vi "Demonstration of k-means assumptions.vi"() -> ()   [LabVIEW 2020]
doc: "This example is meant to illustrate situations where k-means will produce unintuitive and possibly unexpected clusters. In the first three plots, the input data does not conform to some implicit assumption that k-means makes and undesirable clusters are produced as a result. In the last plot, k-means returns intuitive clusters despite unevenly sized blobs."
uses:
  Model/Unsupervised/Cluster/KMeans/KMeans.lvclass
  C:/Users/cipop/TDF Dropbox/2_Technologies de France/1 - Services et Etudes/PLAIY/2 - DEV/PLAIYLAB/code/Model/Model.lvclass
  Model/Unsupervised/Cluster/KMeans/Controls/kmeans_params.ctl
  Display/Classification/2D/Predicted/Controls/PredictedParameter.ctl
  Display/_Controls/Style.ctl
  <vilib>/Analysis/baseanly.llb/Real A x B.vi
  Model/Unsupervised/Cluster/KMeans/KMeans.vi
  <vilib>/Analysis/Matrix/Numeric/Conversions/Array To Matrix - RA2.vi
  <vilib>/Analysis/Matrix/Numeric/Conversions/Matrix To Array - RM.vi
  <vilib>/Analysis/Matrix/NI_Matrix.lvlib
  <vilib>/Analysis/NI_AALBase.lvlib
panel:
  in  "Local":T1
  in  "error in (no error)":errorcluster caption="entrée d'erreur (pas d'erreur)"
  out "error out":errorcluster
  out "Plot 4":cluster{"X":dbl[], "Y":dbl[]}[](graph) caption="Unevenly Sized Blobs"
  out "Plot 3":cluster{"X":dbl[], "Y":dbl[]}[](graph) caption="Unequal Variance"
  out "Plot 2":cluster{"X":dbl[], "Y":dbl[]}[](graph) caption="Anisotropicly Distributed Blobs"
  out "Plot":cluster{"X":dbl[], "Y":dbl[]}[](graph) caption="Incorrect Number of Blobs"
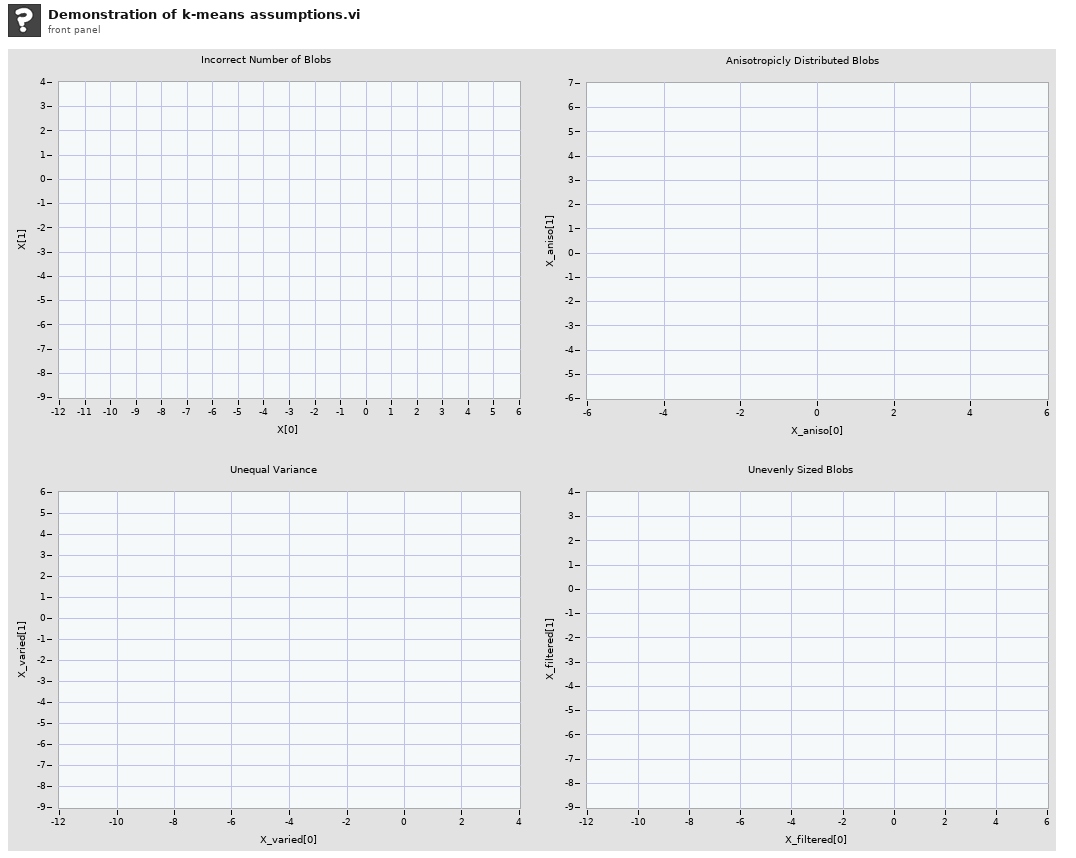
[diagram p1: front panel]
types:
  T1 = cluster{"X":dbl[][], "y":dbl[], "varied":dbl[][], "KMeans":refnum<class "KMeans.lvclass">}
  T2 = cluster{"n_samples":i32[], "n_features":u32, "centers":i32[][], "cluster_std":dbl[], "centermin":dbl, "centermax":dbl, "shuffle":bool, "random_state":i32, "Returns":string}
  T3 = typedef "Style.ctl" = enum16{"Empty circle", "Full circle", "Empty square", "Full square", "Cross"}
  T4 = typedef "PredictedParameter.ctl" = cluster{"Plot":refnum<vi>, "Data":cluster{"X":dbl[][], "Predict":dbl[][]}, "Indexe":cluster{"X":i32, "Y":i32}, "Point Property":cluster{"Style":T3, "Label Color":u32[]}}
  T5 = typedef "kmeans_params.ctl" = cluster{"n_clusters":dbl, "init":cluster{"init_type":string, "init_list":dbl[][]}, "n_init":dbl, "max_iter":dbl, "tol":dbl, "verbose":dbl, "random_state":dbl, "copy_x":bool, "algorithm":string}
  T6 = cluster{" 4DArray":cluster{"1":string[][], "2":string[][]}[], " 3DArray":cluster{"Tableau":string[][]}[], "Sparse Matrix 2DArray":string[][], " 2DArray":string[][], " 1DArray":string[]}
  T7 = typedef "NI_Matrix.lvlib/RealMatrix.ctl" = dbl[][]
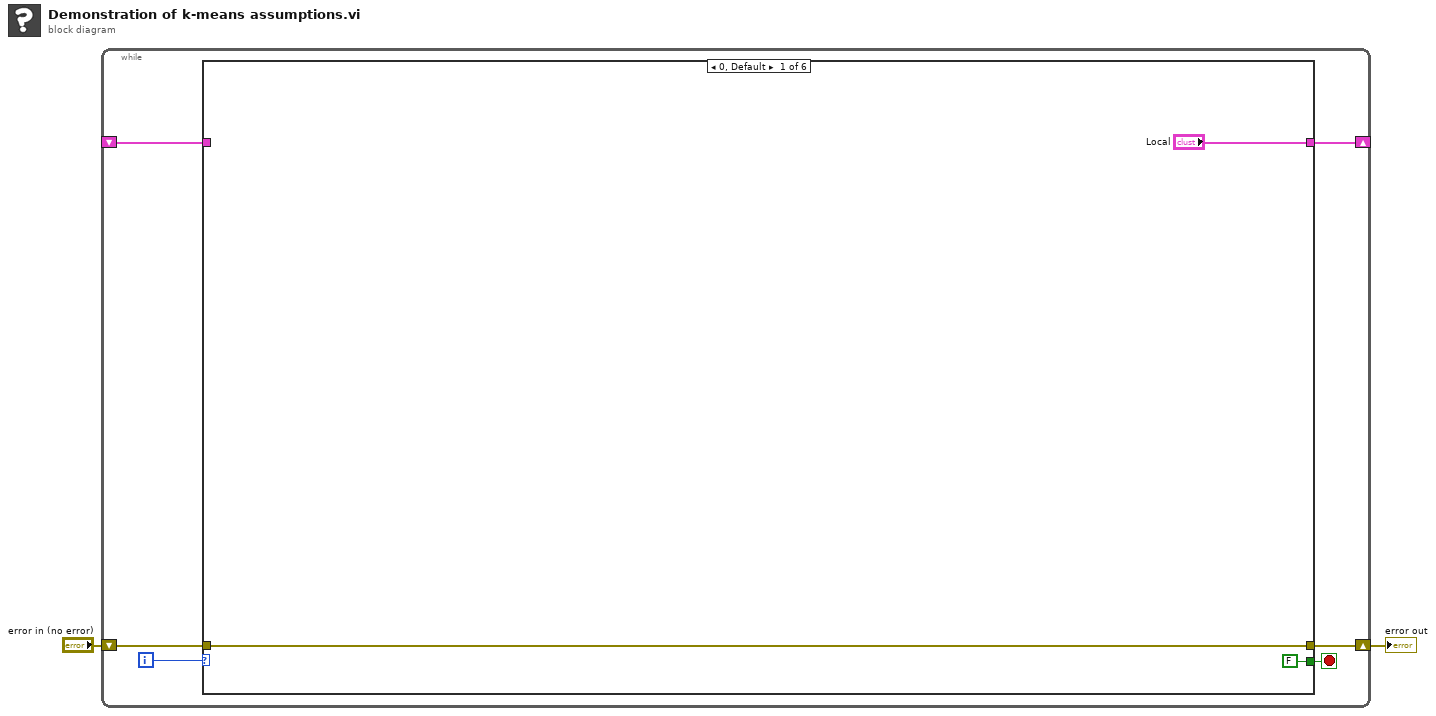
[diagram p0: block diagram]
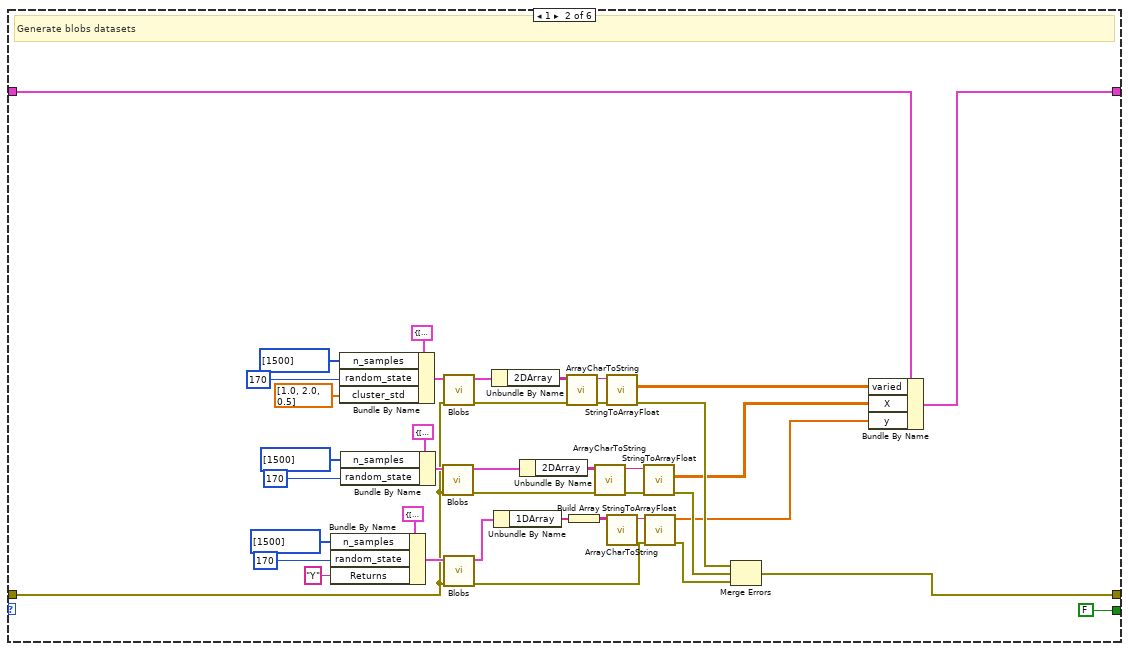
[diagram p2: hidden frame]
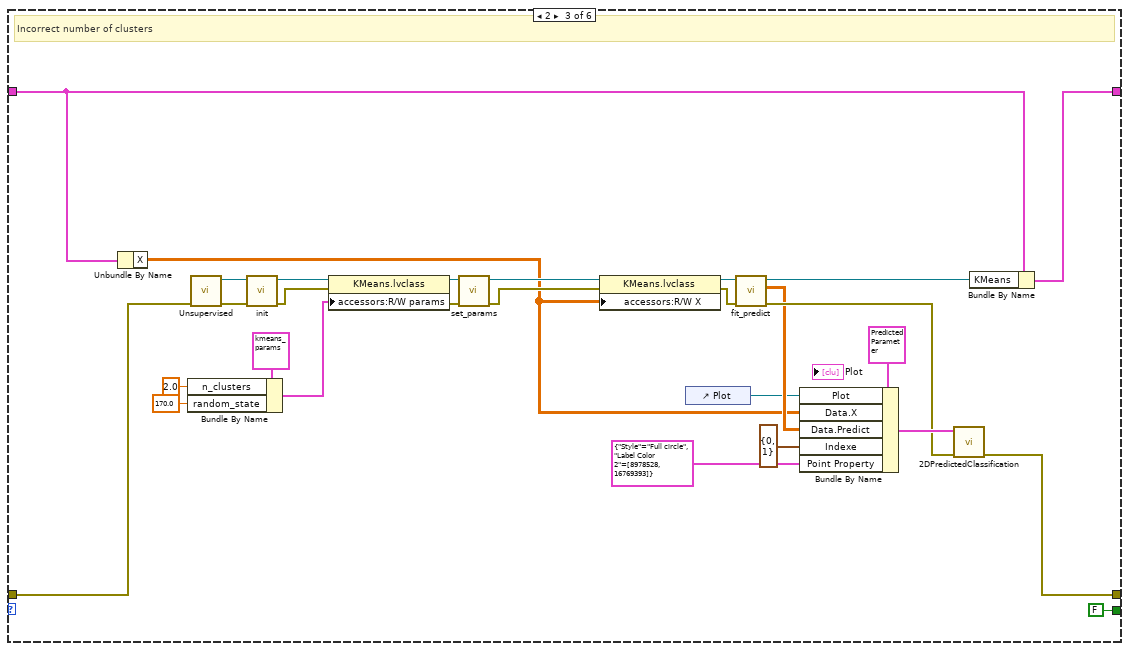
[diagram p3: hidden frame]
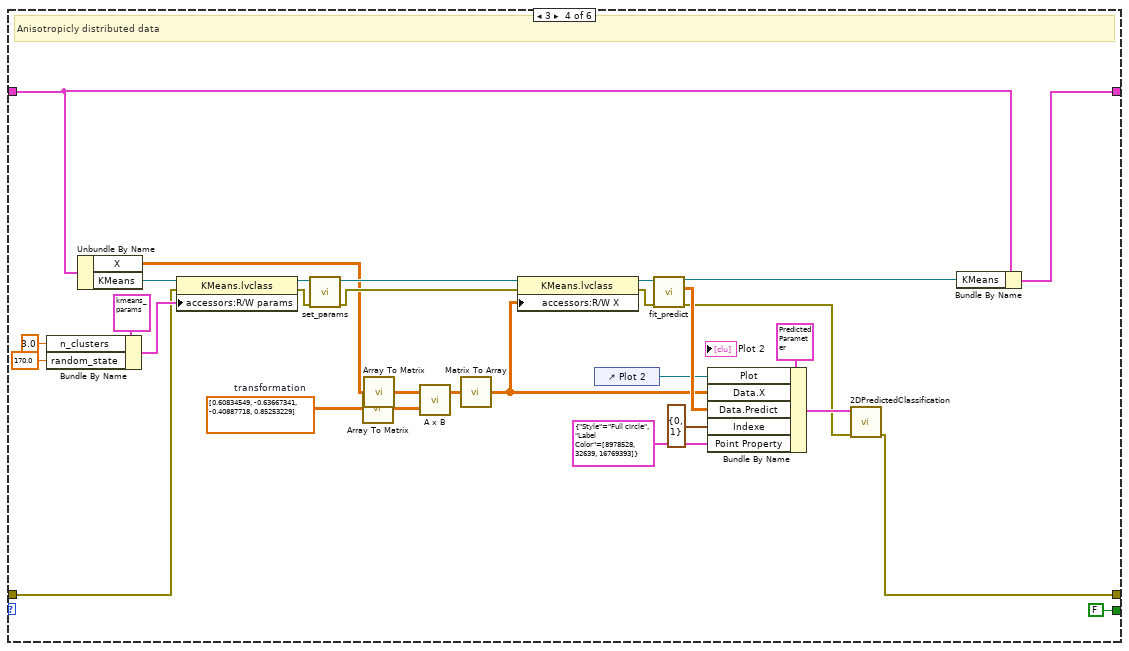
[diagram p4: hidden frame]
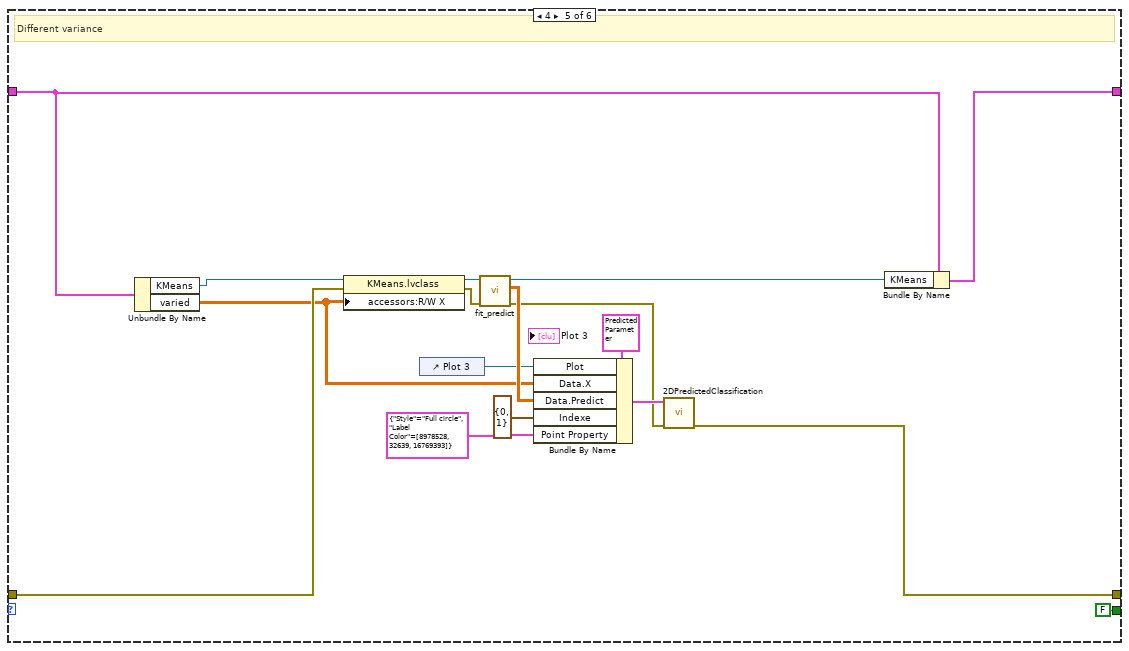
[diagram p5: hidden frame]
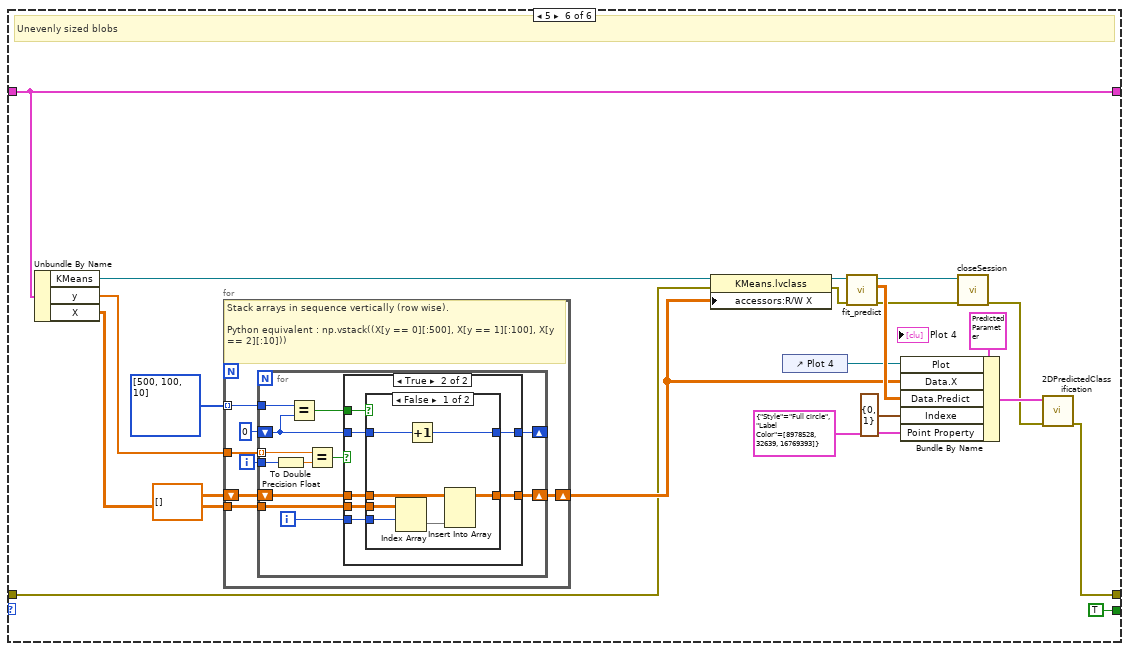
[diagram p6: hidden frame]
diagram:
  n1 = while {
    shift-right: [w6] -> w1
    shift-left: "error in (no error)" -> [w7]
    shift-right: [w4] -> _
    shift-left: _ -> [w3]
    i -> [w8]
    stop <- w5 stop-if-true
    n2 = case shown="0, Default" w8 {
      tunnel: w7 -> [w10 w19 w56 w86 w116 w132]
      tunnel: [w10 w29 w57 w90 w115 w131] -> w6
      tunnel: [FALSE FALSE FALSE FALSE FALSE TRUE] -> w5
      tunnel: ["Local" w15 w51 w79 w110 w125] -> w4
      tunnel: w3 -> [_ w16 w52 w81 w111 w125]
      frame 0, Default {
      }
      frame 1 {
        # "Generate blobs datasets"
        n3 = Bundle By Name(cluster=T2 {"n_samples"=[100], "n_features"=2, "centers"=[], "cluster_std"=[1.0], "centermin"=-10.0, "centermax"=10.0, "shuffle"=TRUE, "random_state"=-1, "Returns"="X"} ("make_blobs"), "n_samples"=i32[] [1500], "random_state"=170, "Returns"="Y") -> (w38:T2)
        n4 = Bundle By Name(cluster=T2 {"n_samples"=[100], "n_features"=2, "centers"=[], "cluster_std"=[1.0], "centermin"=-10.0, "centermax"=10.0, "shuffle"=TRUE, "random_state"=-1, "Returns"="X"} ("make_blobs"), "n_samples"=i32[] [1500], "random_state"=170, "cluster_std"=dbl[] [1.0, 2.0, 0.5]) -> (w21:T2)
        n5 = Bundle By Name(cluster=T2 {"n_samples"=[100], "n_features"=2, "centers"=[], "cluster_std"=[1.0], "centermin"=-10.0, "centermax"=10.0, "shuffle"=TRUE, "random_state"=-1, "Returns"="X"} ("make_blobs"), "n_samples"=i32[] [1500], "random_state"=170) -> (w49:T2)
        n6 = call "Blobs.vi"("error in (no error)"=w19, "make_blobs"=w49) -> ("error out"=w42:errorcluster, "Data"=w45:T6)  [unwired: 8 in]
        n7 = call "Blobs.vi"("error in (no error)"=w19, "make_blobs"=w21) -> ("error out"=w28:errorcluster, "Data"=w25:T6)  [unwired: 8 in]
        n8 = call "Blobs.vi"("error in (no error)"=w19, "make_blobs"=w38) -> ("error out"=w33:errorcluster, "Data"=w34:T6)  [unwired: 8 in]
        n9 = Unbundle By Name(w25) -> ("2DArray"=w27:string[][])
        n10 = Unbundle By Name(w34) -> ("1DArray"=w36:string[])
        n11 = Unbundle By Name(w45) -> ("2DArray"=w43:string[][])
        n12 = call "ArrayCharToString.vi"("TAB"=w27) -> ("Instruction"=w26:string)  [unwired: 10 in]
        n13 = Build Array(w36) -> (w32:string[][])
        n14 = call "ArrayCharToString.vi"("TAB"=w43) -> ("Instruction"=w44:string)  [unwired: 10 in]
        n15 = call "StringToArrayFloat.vi"("entrée d'erreur (pas d'erreur)"=w28, "Return value"=w26) -> ("error IO"=w18:errorcluster, "2DArray"=w14:dbl[][])  [unwired: 7 in, 1 out]
        n16 = call "ArrayCharToString.vi"("TAB"=w32) -> ("Instruction"=w35:string)  [unwired: 10 in]
        n17 = call "StringToArrayFloat.vi"("entrée d'erreur (pas d'erreur)"=w42, "Return value"=w44) -> ("error IO"=w30:errorcluster, "2DArray"=w13:dbl[][])  [unwired: 7 in, 1 out]
        n18 = call "StringToArrayFloat.vi"("entrée d'erreur (pas d'erreur)"=w33, "Return value"=w35) -> ("error IO"=w31:errorcluster, "1DArray"=w12:dbl[])  [unwired: 7 in, 1 out]
        n19 = Merge Errors(w18, w30, w31) -> (w29:errorcluster)
        n20 = Bundle By Name(cluster=w16, "varied"=w14, "X"=w13, "y"=w12) -> (w15:T1)
      }
      frame 2 {
        # "Incorrect number of clusters"
        n21 = Unbundle By Name(w52) -> ("X"=w53:dbl[][])
        n22 = Bundle By Name(cluster=T5 {"n_clusters"=8.0, "init"={"init_type"="k-means++", "init_list"=[]}, "n_init"=10.0, "max_iter"=300.0, "tol"=0.0001, "verbose"=0.0, "random_state"=0.0, "copy_x"=TRUE, "algorithm"="auto"} ("R/W params"), "n_clusters"=2.0, "random_state"=170.0) -> (w65:T5)
        n23 = call-poly "Unsupervised.vi"("error in"=w56) -> ("error out"=w70:errorcluster, "out"=w71:refnum<class "KMeans.lvclass">)  [unwired: 9 in]
        n24 = call-dynamic "init.vi"("error in (no error)"=w70, "Model en entrée"=w71) -> ("error out"=w72:errorcluster, "Model en sortie"=w76:refnum<class "KMeans.lvclass">)  [unwired: 8 in]
        n25 = property class="KMeans.lvclass"(reference=w76, error in=w72, "accessors:R/W params"=w65) -> (reference out=w75:refnum<class "KMeans.lvclass">, error out=w77:errorcluster)
        n26 = call-dynamic "set_params.vi"("error in (no error)"=w77, "KMeans.lvclass 2"=w75) -> ("error out"=w73:errorcluster, "KMeans.lvclass"=w74:refnum<class "KMeans.lvclass">)  [unwired: 8 in]
        n27 = property class="KMeans.lvclass"(reference=w74, error in=w73, "accessors:R/W X"=w53) -> (reference out=w67:refnum<class "KMeans.lvclass">, error out=w66:errorcluster)
        n28 = control-ref of="Plot"() -> (w55:refnum<vi>)
        n29 = call-dynamic "fit_predict.vi"("error in (no error)"=w66, "KMeans.lvclass 2"=w67) -> ("error out"=w61:errorcluster, "C"=w60:dbl[][], "KMeans.lvclass"=w50:refnum<class "KMeans.lvclass">)  [unwired: 7 in]
        n30 = Bundle By Name(cluster=T4 {"Plot"=refnum, "Data"={"X"=[], "Predict"=[]}, "Indexe"={"X"=0, "Y"=1}, "Point Property"={"Style"=enum."Full circle", "Label Color"=[8978528, 4367871, 1985280]}} ("Parameters"), "Plot"=w55, "Data.X"=w53, "Data.Predict"=w60, "Indexe"=cluster{"X":i32, "Y":i32} {"X"=0, "Y"=1}, "Point Property"=cluster{"Style":T3, "Label Color 2":u32[]} {"Style"=enum."Full circle", "Label Color 2"=[8978528, 16769393]}) -> (w63:T4)
        n31 = call "2DPredictedClassification.vi"("error in"=w61, "Parameters"=w63) -> ("error out"=w57:errorcluster)  [unwired: 9 in]
        n32 = Bundle By Name(cluster=w52, "KMeans"=w50) -> (w51:T1)
      }
      frame 3 {
        w106 = dbl[][] [[0.60834549, -0.63667341], [-0.40887718, 0.85253229]]  # transformation
        # "Anisotropicly distributed data"
        n33 = Bundle By Name(cluster=T5 {"n_clusters"=8.0, "init"={"init_type"="k-means++", "init_list"=[]}, "n_init"=10.0, "max_iter"=300.0, "tol"=0.0001, "verbose"=0.0, "random_state"=0.0, "copy_x"=TRUE, "algorithm"="auto"} ("R/W params"), "n_clusters"=3.0, "random_state"=170.0) -> (w89:T5)
        n34 = Unbundle By Name(w81) -> ("X"=w82:dbl[][], "KMeans"=w78:refnum<class "KMeans.lvclass">)
        n35 = property class="KMeans.lvclass"(reference=w78, error in=w86, "accessors:R/W params"=w89) -> (reference out=w99:refnum<class "KMeans.lvclass">, error out=w85:errorcluster)
        n36 = call-dynamic "set_params.vi"("error in (no error)"=w85, "KMeans.lvclass 2"=w99) -> ("error out"=w101:errorcluster, "KMeans.lvclass"=w100:refnum<class "KMeans.lvclass">)  [unwired: 8 in]
        n37 = call-poly <vilib>:"Array To Matrix.vi"("Real 2D Array"=w106) -> ("Real Matrix"=w105:T7)
        n38 = call-poly <vilib>:"Array To Matrix.vi"("Real 2D Array"=w82) -> ("Real Matrix"=w107:T7)
        n39 = call-poly <vilib>:"A x B.vi"("B"=w105, "A"=w107) -> ("A x B"=w104:T7)  [unwired: 1 out]
        n40 = call-poly <vilib>:"Matrix To Array.vi"("Real Matrix"=w104) -> ("Real 2D Array"=w83:dbl[][])
        n41 = property class="KMeans.lvclass"(reference=w100, error in=w101, "accessors:R/W X"=w83) -> (reference out=w102:refnum<class "KMeans.lvclass">, error out=w103:errorcluster)
        n42 = control-ref of="Plot 2"() -> (w87:refnum<vi>)
        n43 = call-dynamic "fit_predict.vi"("error in (no error)"=w103, "KMeans.lvclass 2"=w102) -> ("error out"=w91:errorcluster, "C"=w92:dbl[][], "KMeans.lvclass"=w80:refnum<class "KMeans.lvclass">)  [unwired: 7 in]
        n44 = Bundle By Name(cluster=T4 {"Plot"=refnum, "Data"={"X"=[], "Predict"=[]}, "Indexe"={"X"=0, "Y"=1}, "Point Property"={"Style"=enum."Full circle", "Label Color"=[8978528, 4367871, 1985280]}} ("Parameters"), "Plot"=w87, "Data.X"=w83, "Data.Predict"=w92, "Indexe"=cluster{"X":i32, "Y":i32} {"X"=0, "Y"=1}, "Point Property"=cluster{"Style":T3, "Label Color":u32[]} {"Style"=enum."Full circle", "Label Color"=[8978528, 32639, 16769393]}) -> (w94:T4)
        n45 = call "2DPredictedClassification.vi"("error in"=w91, "Parameters"=w94) -> ("error out"=w90:errorcluster)  [unwired: 9 in]
        n46 = Bundle By Name(cluster=w81, "KMeans"=w80) -> (w79:T1)
      }
      frame 4 {
        # "Different variance"
        n47 = Unbundle By Name(w111) -> ("KMeans"=w108:refnum<class "KMeans.lvclass">, "varied"=w112:dbl[][])
        n48 = property class="KMeans.lvclass"(reference=w108, error in=w116, "accessors:R/W X"=w112) -> (reference out=w124:refnum<class "KMeans.lvclass">, error out=w123:errorcluster)
        n49 = control-ref of="Plot 3"() -> (w114:refnum<vi>)
        n50 = call-dynamic "fit_predict.vi"("error in (no error)"=w123, "KMeans.lvclass 2"=w124) -> ("error out"=w117:errorcluster, "C"=w118:dbl[][], "KMeans.lvclass"=w109:refnum<class "KMeans.lvclass">)  [unwired: 7 in]
        n51 = Bundle By Name(cluster=T4 {"Plot"=refnum, "Data"={"X"=[], "Predict"=[]}, "Indexe"={"X"=0, "Y"=1}, "Point Property"={"Style"=enum."Full circle", "Label Color"=[8978528, 4367871, 1985280]}} ("Parameters"), "Plot"=w114, "Data.X"=w112, "Data.Predict"=w118, "Indexe"=cluster{"X":i32, "Y":i32} {"X"=0, "Y"=1}, "Point Property"=cluster{"Style":T3, "Label Color":u32[]} {"Style"=enum."Full circle", "Label Color"=[8978528, 32639, 16769393]}) -> (w119:T4)
        n52 = call "2DPredictedClassification.vi"("error in"=w117, "Parameters"=w119) -> ("error out"=w115:errorcluster)  [unwired: 9 in]
        n53 = Bundle By Name(cluster=w111, "KMeans"=w109) -> (w110:T1)
      }
      frame 5 {
        # "Unevenly sized blobs"
        n54 = Unbundle By Name(w125) -> ("KMeans"=w128:refnum<class "KMeans.lvclass">, "y"=w126:dbl[], "X"=w127:dbl[][])
        n55 = for {
          tunnel: w126 -> [w152]
          tunnel: w127 -> [w150]
          tunnel: i32[] [500, 100, 10] ("n_samples") -> [w147] mode=indexing
          shift-right: [w149] -> w133
          shift-left: dbl[][] [] ("2DArray") -> [w148]
          i -> [w151]
          # "Stack arrays in sequence vertically (row wise).\n\nPython equivalent : np.vstack((X[y == 0][:500], X[y == 1][:100], X[y == 2][:10]))"
          n56 = for {
            tunnel: w152 -> [w159] mode=indexing
            tunnel: w151 -> [w160]
            tunnel: w150 -> [w163]
            shift-right: [w162] -> w149
            shift-left: w148 -> [w161]
            tunnel: w147 -> [w158]
            shift-right: [w153] -> _
            shift-left: 0 -> [w154]
            i -> [w157]
            n57 = To Double Precision Float(number=w160) -> (double precision float=w164:dbl)
            n58 = Equal?(x=w158, y=w154) -> (x = y?=w155:bool)
            n59 = Equal?(x=w159, y=w164) -> (x = y?=w156:bool)
            n60 = case shown="True" w156 {
              tunnel: w163 -> [_ w173]
              tunnel: w157 -> [_ w172]
              tunnel: [w166 w171] -> w162
              tunnel: w161 -> [w166 w170]
              tunnel: w155 -> [_ w169]
              tunnel: w154 -> [w165 w168]
              tunnel: [w165 w167] -> w153
              frame False {
              }
              frame True {
                n61 = case shown="False" w169 {
                  tunnel: w173 -> [w180 _]
                  tunnel: w172 -> [w179 _]
                  tunnel: [w178 w182] -> w171
                  tunnel: w170 -> [w174 w182]
                  tunnel: w168 -> [w176 w181]
                  tunnel: [w175 w181] -> w167
                  frame False {
                    n62 = Index Array(array=w180, index (row)=w179) -> (element=w177:dbl[])  [unwired: 1 in]
                    n63 = Increment(x=w176) -> (x+1=w175:i32)
                    n64 = Insert Into Array(array=w174, new element=w177) -> (w178:dbl[][])  [unwired: 2 in]
                  }
                  frame True {
                  }
                }
              }
            }
          }
        }
        n65 = property class="KMeans.lvclass"(reference=w128, error in=w132, "accessors:R/W X"=w133) -> (reference out=w134:refnum<class "KMeans.lvclass">, error out=w135:errorcluster)
        n66 = control-ref of="Plot 4"() -> (w130:refnum<vi>)
        n67 = call-dynamic "fit_predict.vi"("error in (no error)"=w135, "KMeans.lvclass 2"=w134) -> ("error out"=w140:errorcluster, "C"=w143:dbl[][], "KMeans.lvclass"=w139:refnum<class "KMeans.lvclass">)  [unwired: 7 in]
        n68 = Bundle By Name(cluster=T4 {"Plot"=refnum, "Data"={"X"=[], "Predict"=[]}, "Indexe"={"X"=0, "Y"=1}, "Point Property"={"Style"=enum."Full circle", "Label Color"=[8978528, 4367871, 1985280]}} ("Parameters"), "Plot"=w130, "Data.X"=w133, "Data.Predict"=w143, "Indexe"=cluster{"X":i32, "Y":i32} {"X"=0, "Y"=1}, "Point Property"=cluster{"Style":T3, "Label Color":u32[]} {"Style"=enum."Full circle", "Label Color"=[8978528, 32639, 16769393]}) -> (w142:T4)
        n69 = call-dynamic "closeSession.vi"("error in"=w140, "Python en entrée"=w139) -> ("error out"=w141:errorcluster)  [unwired: 8 in, 1 out]
        n70 = call "2DPredictedClassification.vi"("error in"=w141, "Parameters"=w142) -> ("error out"=w131:errorcluster)  [unwired: 9 in]
      }
    }
  }
  "error out" <- w1
